vi "DestroyModule.vi"(8 "error in (no error)":errorcluster, 11 "JQMHModule in":refnum<class "RQMHModule.lvclass">) -> (0 "error out":errorcluster)   [LabVIEW 2024, in "RQMHModule.lvclass"]
uses:
  RQMHModule.lvclass
  RQMHModule.lvclass/RQMHModule.ctl
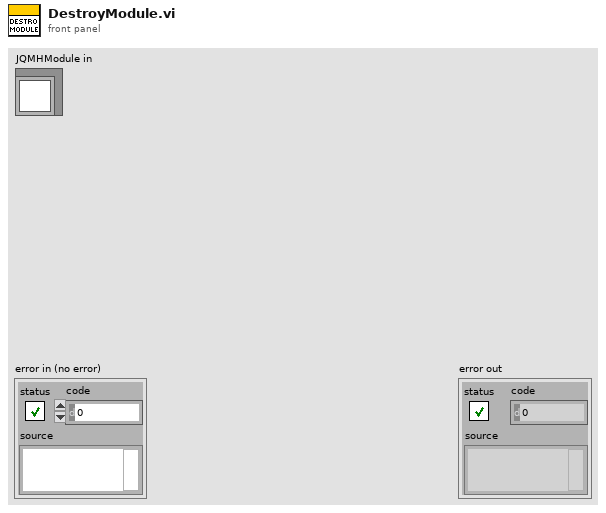
[diagram p1: front panel]
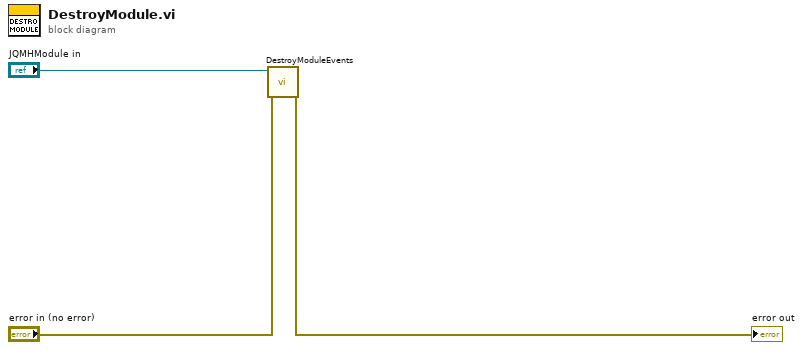
[diagram p0: block diagram]
diagram:
  n1 = call "DestroyModuleEvents.vi"("error in (no error)"="error in (no error)", "JQMHModule in"="JQMHModule in") -> ("error out"=→"error out":errorcluster)  [unwired: 8 in, 1 out]
